vi "Auto-Refresh Read.vi"(8 "error in (no error)":errorcluster, 11 "MSX-E3711 in":refnum<class "MSX-E3711.lvclass">) -> (0 "error out":errorcluster, 1 "Control Data":T1, 2 "1 Sample":T2, 3 "MSX-E3711 out":refnum<class "MSX-E3711.lvclass">)   [LabVIEW 2014, in "MSX-E3711.lvlib" / "MSX-E3711.lvclass"]
uses:
  MSX-E3711.lvclass
  DriverMasterSync/build/DriverMasterSync.lvlibp/APIs/Data Queue/Acquisition Data 1 Sample Cluster.ctl
  DriverMasterSync/build/DriverMasterSync.lvlibp/APIs/Data Queue/Control Data Cluster.ctl
  MSX-E3711.lvclass/MSX-E3711.ctl
  API/MSX-E3711_dll.lvlib
  DriverMasterSync/build/DriverMasterSync.lvlibp/Modules/HAL/DriverMasterSync/DriverMasterSyncClass/DriverMasterSync.lvclass
  DriverMasterSync/build/DriverMasterSync.lvlibp/APIs/Data Queue/WINFAS 2 Data Queue.lvlib
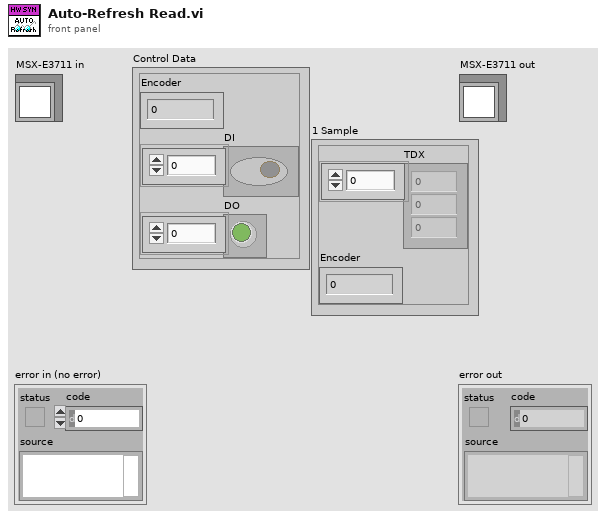
[diagram p1: front panel]
types:
  T1 = typedef "DriverMasterSync.lvlibp/WINFAS 2 Data Queue.lvlib/Control Data Cluster.ctl" = cluster{"Encoder":sgl, "DI":bool[], "DO":bool[]}
  T2 = typedef "DriverMasterSync.lvlibp/WINFAS 2 Data Queue.lvlib/Acquisition Data 1 Sample Cluster.ctl" = cluster{"TDX":sgl[], "Encoder":sgl}
  T3 = typedef "MSX-E3711_dll.lvlib/Connection Data.ctl" = cluster{"MX371x refnum":refnum<k24>, "IP":string, "Connection ID ":refnum<k5>, "MXCommon refnum":refnum<k24>}
  T4 = typedef "MSX-E3711_dll.lvlib/Config Data.ctl" = cluster{"Auto Refresh":cluster{"Average Mode":u64, "Average Value":u64, "Trigger Mask":u64, "Trigger Mode":u64, "Hardware Trigger Edge":u64, "Hardware Trigger Count":u64, "By Trigger Nbr Of Seq To Acquire":u64, "Time stamp":bool, "Analog Output(mm)":bool, "Invert value":bool, "Temperature value":bool, "Incremental counter value":bool, "Diff. mode":bool}, "Gain":sgl[], "Offset":sgl[], "Index":u64, "Range":sgl, "Sequence":cluster{"Nbr Of Sequence":u64, "Nbr Max Sequence To Transfer":u64, "Delay Mode":u64, "Delay Time Unit":u64, "Delay Value":u64, "Trigger Mask":u64, "Trigger Mode":u64, "Hardware Trigger Edge":u64, "Hardware Trigger Count":u64, "By Trigger Nbr Of Seq To Acquire":u64, "Time stamp":bool, "Sequence counter information":bool, "Analog Output(mm)":bool, "Invert value":bool, "Temperature value":bool, "Incremental counter value":bool, "Diff. mode":bool}, "Enable DIO":bool, "IncCounter":cluster{"CounterMode":string, "CounterOptionDIRECT  ":bool, "CounterOptionOthers":bool, "CounterClear ":bool, "Cantidad de Pulsos":sgl, "Reducción":sgl}, "IncTemperature":cluster{"ConnectedTempSensor":string, "ConvertMode":string, "InitGainSelection":string, "FrequencySelection":string, "PowerSaveMode":bool, "GainSelection":string, "RefValue":dbl}}
  T5 = typedef "MSX-E3711_dll.lvlib/Adquisition Data.ctl" = cluster{"Adq. Sequence":cluster{"Adquisition Value":u32[][], "Counter Value":u32[], "TSs - TSu - NAS":u64[][], "Status IO Port":bool[]}, "Adq. Auto Refresh":cluster{"Adquisition Value":u64[], "Status IO Port":bool[], "Counter value":u32}}
  T6 = cluster{"Adquisition Value":u64[], "Status IO Port":bool[], "Counter value":u32}
  T7 = typedef "DriverMasterSync.lvlibp/HAL Config Data.ctl" = cluster{"HWSync Index":u32, "Driver Name":string, "Channel Mask":u64}
  T8 = typedef "DriverMasterSync.lvlibp/WINFAS 2 Data Queue.lvlib/Acquisition Data Cluster.ctl" = T2[]
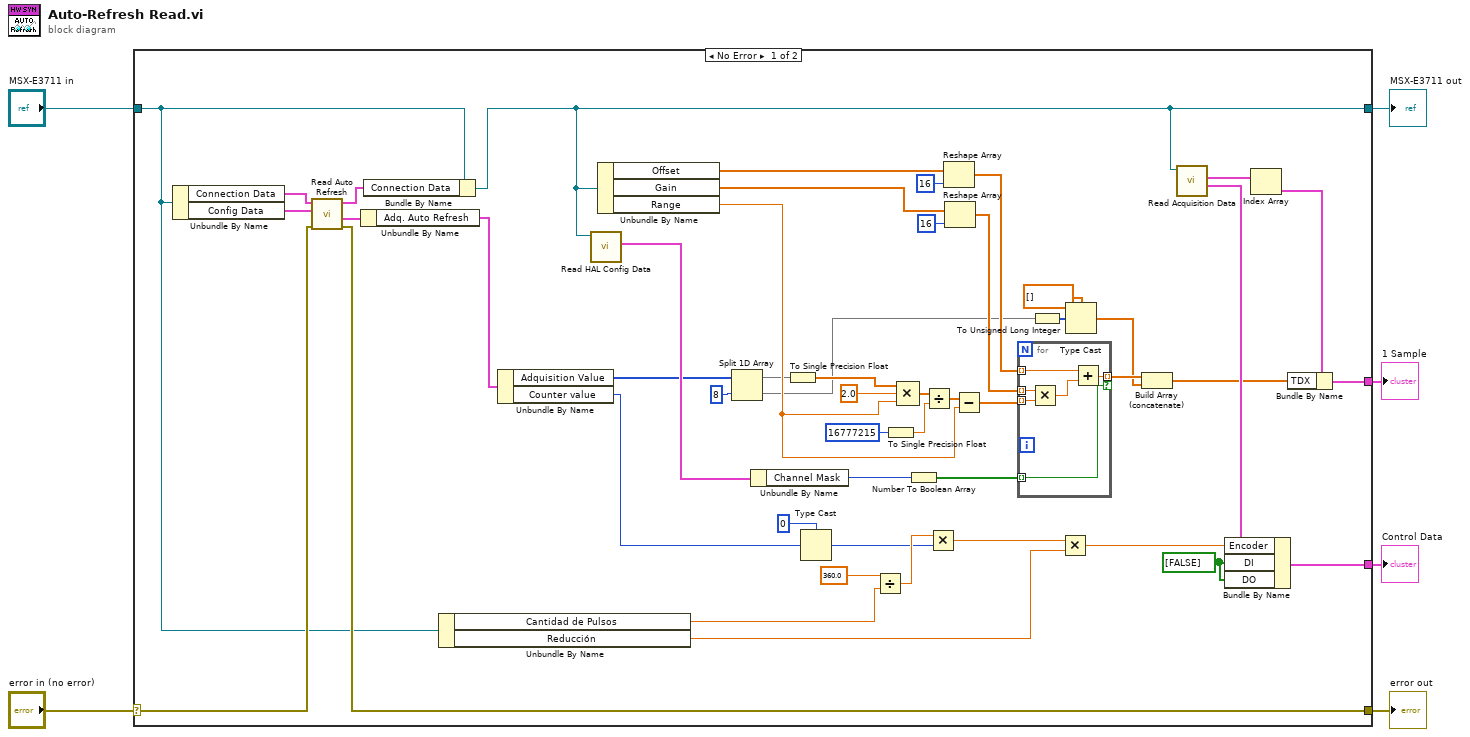
[diagram p0: block diagram]
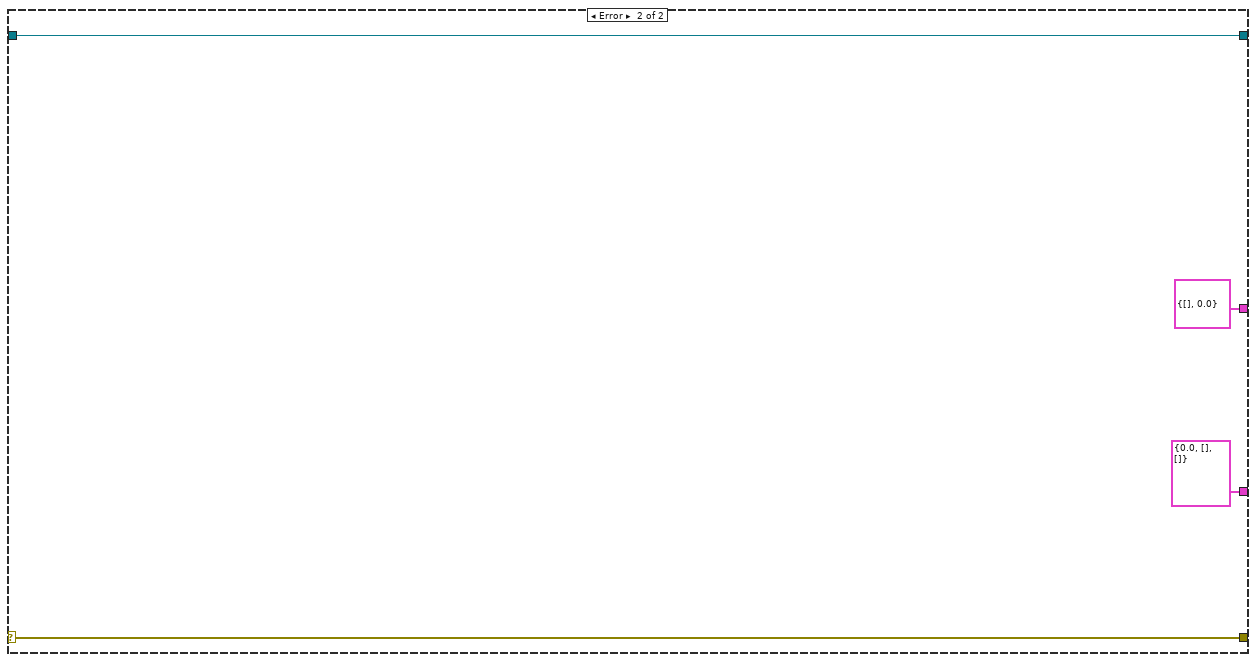
[diagram p2: hidden frame]
diagram:
  n1 = case shown="No Error" "error in (no error)" {
    selector: "error in (no error)" -> [w38 w66]
    tunnel: [w37 w66] -> w5
    tunnel: [w33 w65] -> w3
    tunnel: "MSX-E3711 in" -> [w16 w65]
    tunnel: [w30 T1 {"Encoder"=0.0, "DI"=[], "DO"=[]} ("Control Data")] -> w1
    tunnel: [w29 T2 {"TDX"=[], "Encoder"=0.0} ("1 Sample")] -> w2
    frame No Error {
      w17 = bool[] [FALSE] ("DI")
      n2 = Unbundle By Name(w16) -> ("Connection Data"=w39:T3, "Config Data"=w28:T4)
      n3 = call "Read Auto Refresh.vi"("error in (no error)"=w38, "Config Data"=w28, "Connection Data In"=w39) -> ("error out"=w37:errorcluster, "Adquisition Data Out"=w35:T5, "Connection Data Out"=w36:T3)  [unwired: 6 in]
      n4 = Unbundle By Name(w35) -> ("Adq. Auto Refresh"=w55:T6)
      n5 = Bundle By Name(cluster=w16, "Connection Data"=w36) -> (w33:refnum<class "MSX-E3711.lvclass">)
      n6 = Unbundle By Name(w16) -> ("Cantidad de Pulsos"=w12:sgl, "Reducción"=w11:sgl)
      n7 = Unbundle By Name(w55) -> ("Adquisition Value"=w23:u64[], "Counter value"=w9:u32)
      n8 = call "Read HAL Config Data.vi"("DriverMasterSync in"=w33) -> ("HAL Config Data"=w34:T7)  [unwired: 8 in, 2 out]
      n9 = Unbundle By Name(w33) -> ("Offset"=w54:sgl[], "Gain"=w51:sgl[], "Range"=w41:sgl)
      n10 = Split 1D Array(array=w23, index=8) -> (first subarray=w22:u64[], second subarray=w20:u64[])
      n11 = Unbundle By Name(w34) -> ("Channel Mask"=w48:u64)
      n12 = To Single Precision Float(number=w22) -> (single precision float=w21:sgl[])
      n13 = Type Cast(type=0, x=w9) -> (*(type *) &x=w7:i32)
      n14 = Divide(x=sgl 360.0 ("y"), y=w12) -> (x/y=w14:sgl)
      n15 = To Single Precision Float(number=u64 16777215 ("x")) -> (single precision float=w45:sgl)
      n16 = Compound Arithmetic op=MULTIPLY(w21, sgl 2.0 ("x"), w41) -> (w44:sgl[])
      n17 = Number To Boolean Array(number=w48) -> (Boolean array=w47:bool[])
      n18 = Divide(x=w44, y=w45) -> (x/y=w43:sgl[])
      n19 = Multiply(x=w14, y=w7) -> (x*y=w13:sgl)
      n20 = Reshape Array(w54, 16 ("dimension size")) -> (w49:sgl[])
      n21 = Reshape Array(w51, 16 ("dimension size")) -> (w50:sgl[])
      n22 = Subtract(x=w43, y=w41) -> (x-y=w40:sgl[])
      n23 = for {
        tunnel: w50 -> [w62] mode=indexing
        tunnel: w49 -> [w61] mode=indexing
        tunnel: w40 -> [w59] mode=indexing
        tunnel: [w58] -> w25 mode=indexing if=w57
        tunnel: w47 -> [w57] mode=indexing
        n24 = Multiply(x=w62, y=w59) -> (x*y=w60:sgl)
        n25 = Add(x=w61, y=w60) -> (x+y=w58:sgl)
      }
      n26 = To Unsigned Long Integer(number=w20) -> (unsigned 32bit integer=w24:u32[])
      n27 = Multiply(x=w13, y=w11) -> (x*y=w10:sgl)
      n28 = Type Cast(type=sgl[] [], x=w24) -> (*(type *) &x=w19:sgl[])
      n29 = Build Array (concatenate)(w25, w19) -> (w26:sgl[])
      n30 = call "Read Acquisition Data.vi"("DriverMasterSync in"=w33) -> ("Control Data"=w31:T1, "Acquisition Data"=w32:T8)  [unwired: 7 in, 2 out]
      n31 = Bundle By Name(cluster=w31, "Encoder"=w10, "DI"=w17, "DO"=w17) -> (w30:T1)
      n32 = Index Array(array=w32) -> (element=w56:T2)  [unwired: 1 in]
      n33 = Bundle By Name(cluster=w56, "TDX"=w26) -> (w29:T2)
    }
    frame Error {
    }
  }
  "error out" <- w5
  "MSX-E3711 out" <- w3
  "1 Sample" <- w2
  "Control Data" <- w1
